vi "条件结束.vi"() -> ()   [LabVIEW 2020]
doc: "本VI是为《我和LabVIEW》一书编写的示例。\n关于本书的介绍请参考网页：\nhttp://ruanqizhen.spaces.live.com/blog/cns!5852D4F797C53FB6!4310.entry"
panel:
  out "数值":i32
  in  "字符串":string
  in  "数组":string[](array[string])
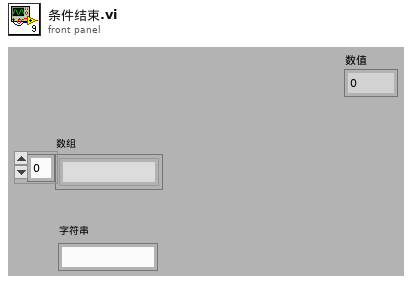
[diagram p1: front panel]
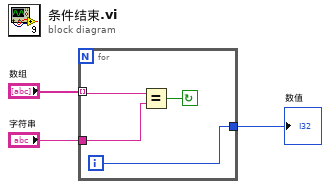
[diagram p0: block diagram]
diagram:
  n1 = for {
    tunnel: "数组" -> [w7] mode=indexing
    tunnel: "字符串" -> [w6]
    tunnel: [w4] -> w1
    i -> [w4]
    stop <- w5 continue-if-true
    n2 = Equal?(x=w7, y=w6) -> (x = y?=w5:bool)
  }
  "数值" <- w1
